vi "limit_sym.vi"(6 "Limit":dbl, 11 "Input":dbl) -> (2 "Output":dbl)   [LabVIEW 2025]
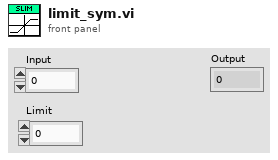
[diagram p1: front panel]
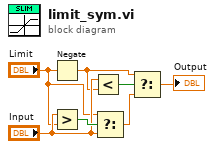
[diagram p0: block diagram]
diagram:
  n1 = Negate(x="Limit") -> (-x=w1:dbl)
  n2 = Greater?(x="Input", y="Limit") -> (0:w6:bool)
  n3 = Less?(x="Input", y=w1) -> (x < y?=w5:bool)
  n4 = Select(t="Limit", s=w6, f="Input") -> (s? t:f=w4:dbl)
  n5 = Select(t=w1, s=w5, f=w4) -> (s? t:f=→"Output":dbl)
